vi "Notes to ITX.vi"(1 "Notes":string) -> (0 "ITX Notes":string)   [LabVIEW 2016, in "LV to ITX.lvclass"]
uses:
  LV to ITX.lvclass
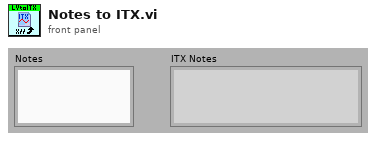
[diagram p1: front panel]
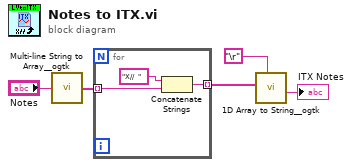
[diagram p0: block diagram]
diagram:
  n1 = call <userlib>:"Multi-line String to Array__ogtk.vi"("string"="Notes") -> ("lines"=w1:string[])
  n2 = for {
    tunnel: w1 -> [w7] mode=indexing
    tunnel: [w6] -> w3 mode=indexing
    n3 = Concatenate Strings("X//  " ("string"), w7) -> (w6:string)
  }
  n4 = call <userlib>:"1D Array to String__ogtk.vi"("delimiter (Tab)"="\r", "Array of Strings"=w3) -> ("delimited string"=→"ITX Notes":string)  [unwired: 9 in]
